vi "Runout.vi"(8 "error in":errorcluster, 11 "Data In":T3) -> (0 "error out":errorcluster, 3 "Data Out":T3)   [LabVIEW 2025]
uses:
  Controls/Wheel_data.ctl
  Controls/Spork plot.ctl
  Controls/Spoke_stats.ctl
  Controls/Spork type.ctl
  Controls/Tension.ctl
  Controls/Tension_Output.ctl
  Controls/Runout.ctl
  Controls/Runout Output.ctl
  Controls/Nippel Turn Direction.ctl
  Controls/Aditional Info.ctl
panel:
  out "Runout Graph":cluster{dbl[], dbl[]}[](graph)
  in  "Measure":bool
  out "Spoke":i32[](array[numeric])
  in  "Exit Runout":bool
  out "Std Div":dbl
  out "Avg":dbl
  out "Min Runout":dbl
  out "Max Runout":dbl
  out "Runout Output":T1[](array[typedef])
  in  "Variance":dbl min=0.0 max=25.0 step=5.0 format="%.0f %%"
  out "Last connected to":string
  in  "VISA resource name":refnum<visa-resource-name>
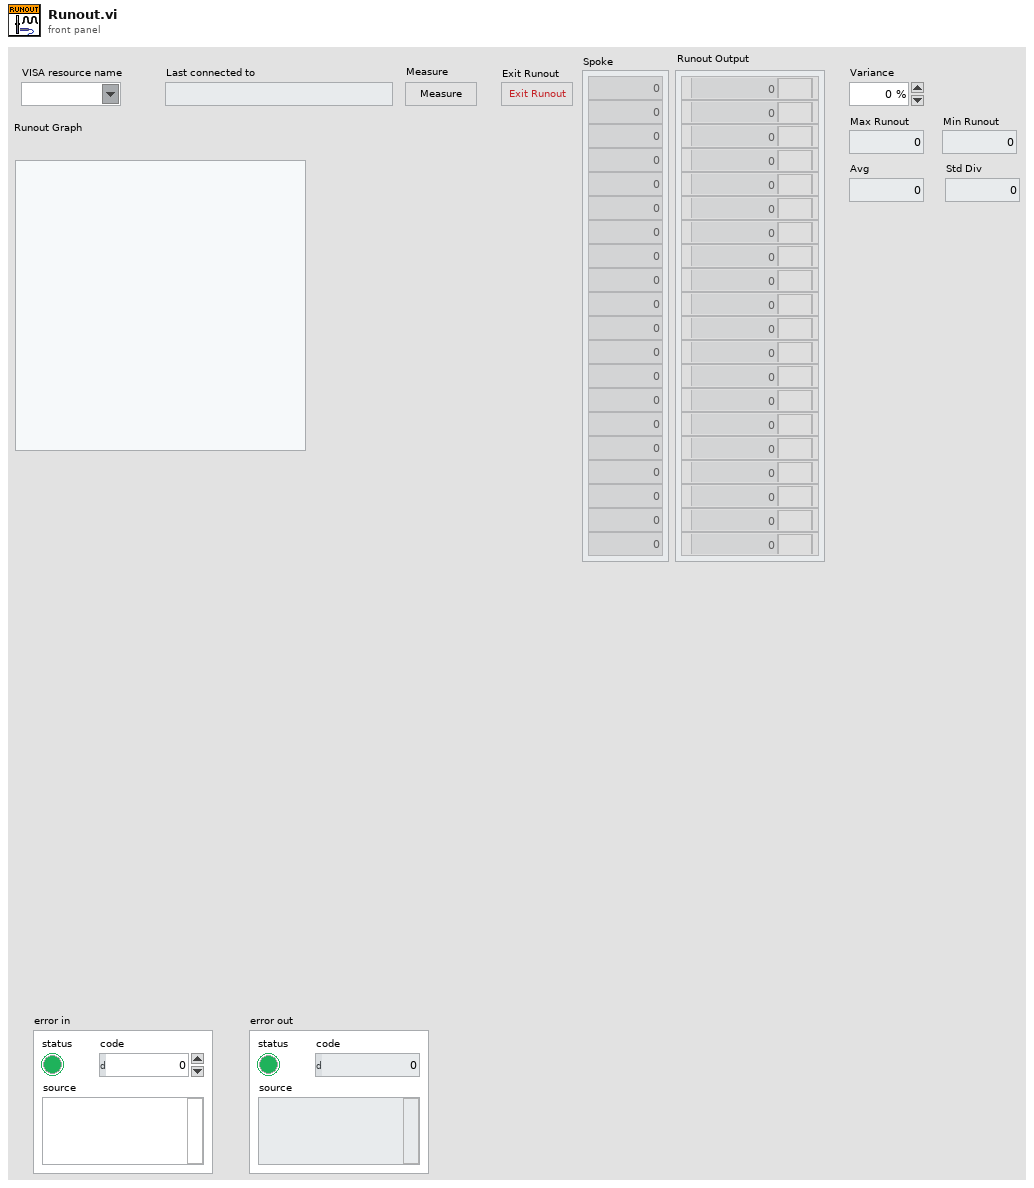
[diagram p1: front panel]
types:
  T1 = typedef "Runout Output.ctl" = cluster{"Value":dbl, "Nippel Direction":T2}
  T2 = typedef "Nippel Turn Direction.ctl" = u16
  T3 = typedef "Wheel_data.ctl" = cluster{"Wheel Grapth":T4[], "Spokes":T5, "Tension":T7, "Runout":T9, "Avaliable Printers":string[], "Aditional Info":T10}
  T4 = typedef "Spork plot.ctl" = cluster{"X":dbl[], "Y":dbl[]}
  T5 = typedef "Spoke_stats.ctl" = cluster{"Spokes number":i32, "Spokes crosses":i32, "Spokes Type":T6}
  T6 = typedef "Spork type.ctl" = enum16{"Steel 1.4mm", "Steel 1.5mm", "Steel 1.6mm", "Steel 1.7mm", "Steel 1.8mm", "Steel 2mm", "Steel 2.3mm", "Steel 2.5mm", "Steel 2.6mm", "Aluminum 2.28mm", "Aluminum 2.54mm", "Aluminum 2.8mm", "Aluminum 3.3mm"}
  T7 = typedef "Tension.ctl" = cluster{"Spokes Tension Left":dbl[], "Tension Graph":T4[], "Average Left":dbl, "Variance":dbl, "Std Div Left":dbl, "Average Right":dbl, "Std Div Right":dbl, "Tension Output Left":T8[], "Tension Output Right":T8[], "Spokes Tension Right":dbl[]}
  T8 = typedef "Tension_Output.ctl" = cluster{"Tenction [kgf]":dbl, "Within Limit":bool}
  T9 = typedef "Runout.ctl" = cluster{"Runout Output":T1[], "Runout Graph":T4[], "Average":dbl, "Std Div":dbl, "Spoke Measured":i32[]}
  T10 = typedef "Aditional Info.ctl" = cluster{"Name":string, "Rims":string, "Hub":string, "Notes":string, "Spokes":string, "Type":enum32{"Item 0", "Item 1"}, "Mechanic's Name":string}
  T11 = typedef "Spoke_side.ctl" = u16
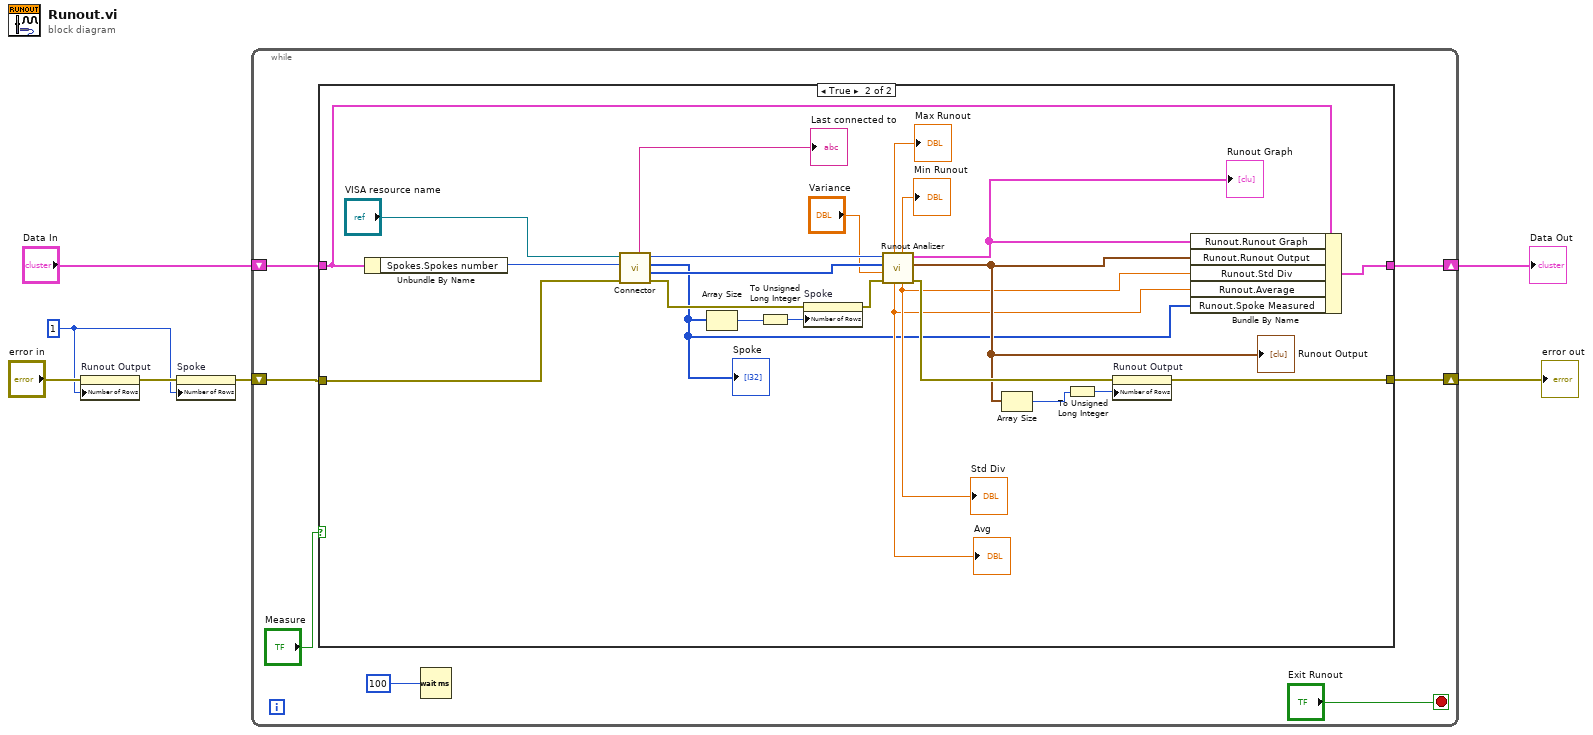
[diagram p0: block diagram]
diagram:
  w1 = u32 1 ("Number of Rows")
  n1 = property on="Runout Output" class="Arr (strict)"(error in="error in", "Number of Rows"=w1) -> (error out=w2:errorcluster)  [unwired: 1 in, 1 out]
  n2 = property on="Spoke" class="Arr (strict)"(error in=w2, "Number of Rows"=w1) -> (error out=w3:errorcluster)  [unwired: 1 in, 1 out]
  n3 = while {
    shift-right: [w13] -> w7
    shift-left: w3 -> [w14]
    shift-right: [w10] -> w5
    shift-left: "Data In" -> [w12]
    stop <- "Exit Runout" stop-if-true
    n4 = case shown="True" "Measure" {
      tunnel: w14 -> [w16 w40]
      tunnel: [w16 w31] -> w13
      tunnel: w12 -> [w15 w26]
      tunnel: [w15 w27] -> w10
      frame False {
      }
      frame True {
        n5 = Unbundle By Name(w26) -> ("Spokes.Spokes number"=w39:i32)
        n6 = call "Connector.vi"("error in"=w40, "Sporks number"=w39, "VISA resource name"="VISA resource name") -> ("error out"=w22:errorcluster, "Measurement"=w35:i32[], "Spoke"=w18:i32[], "First spoke side"=w36:T11, "Instrument IDN"=→"Last connected to":string)  [unwired: 4 in]
        "Spoke" <- w18
        n7 = Array Size(array=w18) -> (size(s)=w20:i32)
        n8 = To Unsigned Long Integer(number=w20) -> (unsigned 32bit integer=w19:u32)
        n9 = property on="Spoke" class="Arr (strict)"(error in=w22, "Number of Rows"=w19) -> (error out=w21:errorcluster)  [unwired: 1 in, 1 out]
        n10 = call "Runout Analizer.vi"("error in"=w21, "Variance"="Variance", "Measurement"=w35, "Side of first spoke"=w36) -> ("error out"=w30:errorcluster, "Runout Output"=w25:T1[], "Polar Graph"=w17:cluster{dbl[], dbl[]}[], "Std Div"=w24:dbl, "Min Runout"=→"Min Runout":dbl, "Avg"=w23:dbl, "Max Runout"=→"Max Runout":dbl)  [unwired: 1 in]
        "Runout Output" <- w25
        "Avg" <- w23
        "Std Div" <- w24
        "Runout Graph" <- w17
        n11 = Array Size(array=w25) -> (size(s)=w28:i32)
        n12 = To Unsigned Long Integer(number=w28) -> (unsigned 32bit integer=w29:u32)
        n13 = property on="Runout Output" class="Arr (strict)"(error in=w30, "Number of Rows"=w29) -> (error out=w31:errorcluster)  [unwired: 1 in, 1 out]
        n14 = Bundle By Name(cluster=w26, "Runout.Runout Graph"=w17, "Runout.Runout Output"=w25, "Runout.Std Div"=w24, "Runout.Average"=w23, "Runout.Spoke Measured"=w18) -> (w27:T3)
      }
    }
    n15 = Wait (ms)(milliseconds to wait=u32 100) -> ()  [unwired: 1 out]
  }
  "Data Out" <- w5
  "error out" <- w7
